vi "dataAcq_get_spectrum.vi"(0 "reference":refnum<class "OSA300.lvclass">, 5 "error in (no error)":errorcluster, 9 "x data create":bool) -> (14 "duplicate reference":refnum<class "OSA300.lvclass">, 19 "error out":errorcluster)   [LabVIEW 2010, in "OSA300.lvclass"]
doc: "Reads data from spectrometer and updates labview buffer spectrum Y array, X is either equidistant, (x min and max), or contains a full X-array. See buffer_get.vi for labview buffer data access.\n\nX: periods/cm\nY: mW absolute pwr, (pwr/resolution)"
uses:
  OSA300.lvclass
  OSA.lvclass
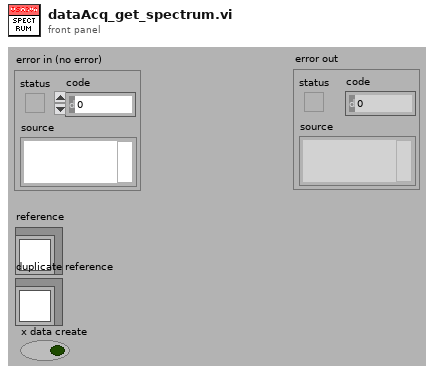
[diagram p1: front panel]
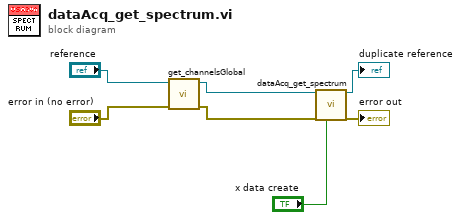
[diagram p0: block diagram]
diagram:
  n1 = call "get_channelsGlobal.vi"("error in (no error)"="error in (no error)", "OSA300 in"="reference") -> ("error out"=w2:errorcluster, "OSA300 out"=w1:refnum<class "OSA300.lvclass">)  [unwired: 8 in]
  n2 = call-parent "dataAcq_get_spectrum.vi"("reference"=w1, "error in (no error)"=w2, "x data create"="x data create") -> ("duplicate reference"=→"duplicate reference":refnum<class "OSA300.lvclass">, "error out"=→"error out":errorcluster)  [unwired: 15 in]
